vi "AnalysatorStringLaden.vi"(11 "Array (Eingang)":string[][](array[string])) -> (2 "string array":string[][](array[string]), 3 "Cluster Array (Ausgang)":T1[](array[typedef]))   [LabVIEW 2020, in "System Einstellungen V2.lvlib"]
uses:
  System Einstellungen V2.lvlib
  AnalysatorDefinition.ctl
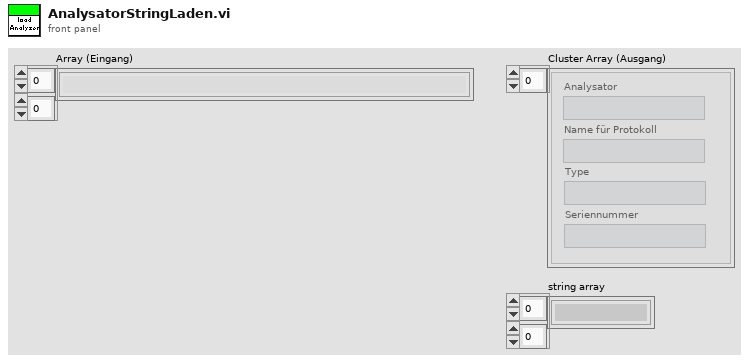
[diagram p1: front panel]
types:
  T1 = typedef "System Einstellungen V2.lvlib/AnalysatorDefinition.ctl" = cluster{"Analysator":string, "Name für Protokoll":string, "Type":string, "Seriennummer":string}
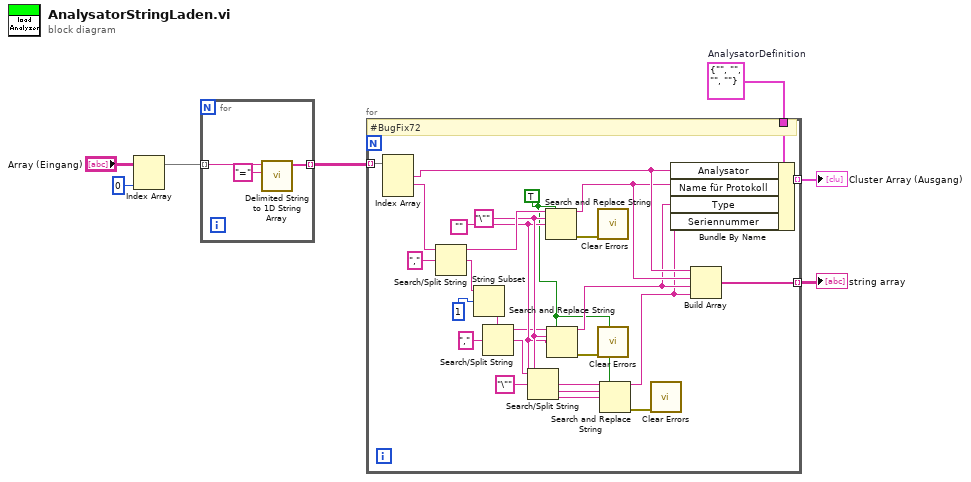
[diagram p0: block diagram]
diagram:
  w6 = T1 {"Analysator"="", "Name für Protokoll"="", "Type"="", "Seriennummer"=""}  # AnalysatorDefinition
  n1 = Index Array(array="Array (Eingang)", index (col)=0 ("Deaktivierter Index (Spalte)")) -> (element=w4:string[])  [unwired: 1 in]
  n2 = for {
    tunnel: w4 -> [w10] mode=indexing
    tunnel: [w8] -> w3 mode=indexing
    n3 = call <vilib>:"Delimited String to 1D String Array.vi"("delimiter"="=", "delimited string"=w10) -> ("string array"=w8:string[])  [unwired: 9 in]
  }
  n4 = for {
    tunnel: w3 -> [w34] mode=indexing
    tunnel: w6 -> [w35]
    tunnel: [w33] -> w7 mode=indexing
    tunnel: [w29] -> w2 mode=indexing
    w16 = ""
    w15 = TRUE ("Alle ersetzen? (F)")
    w17 = "\"" ("Such-String")
    # "#BugFix72"
    n5 = Index Array(array=w34) -> (element #1=w31:string, element #2=w28:string)  [unwired: 3 in, 1 out]
    n6 = Search/Split String(string=w28, search string/char (-)="," ("Such-String/-Zeichen (-)")) -> (substring before match=w26:string, match + rest of string=w24:string)  [unwired: 1 in, 1 out]
    n7 = String Subset(string=w24, offset (0)=1 ("Offset (0)")) -> (substring=w12:string)  [unwired: 1 in]
    n8 = Search/Split String(string=w12, search string/char (-)="," ("Such-String/-Zeichen (-)")) -> (substring before match=w14:string, match + rest of string=w20:string)  [unwired: 1 in, 1 out]
    n9 = Search/Split String(string=w20, search string/char (-)="\"" ("Such-String/-Zeichen (-)")) -> (match + rest of string=w18:string)  [unwired: 1 in, 2 out]
    n10 = Search and Replace String(replace all?=w15, input string=w26, search string=w17, replace string=w16) -> (result string=w30:string, error out=w32:errorcluster)  [unwired: 4 in, 2 out]
    n11 = Search and Replace String(replace all?=w15, input string=w14, search string=w17, replace string=w16) -> (result string=w22:string, error out=w23:errorcluster)  [unwired: 4 in, 2 out]
    n12 = call <vilib>:"Clear Errors.vi"("error in (no error)"=w32) -> ()  [unwired: 5 in, 2 out]
    n13 = call <vilib>:"Clear Errors.vi"("error in (no error)"=w23) -> ()  [unwired: 5 in, 2 out]
    n14 = Search and Replace String(replace all?=w15, input string=w18, search string=w17, replace string=w16) -> (result string=w13:string, error out=w19:errorcluster)  [unwired: 4 in, 2 out]
    n15 = call <vilib>:"Clear Errors.vi"("error in (no error)"=w19) -> ()  [unwired: 5 in, 2 out]
    n16 = Bundle By Name(cluster=w35, "Analysator"=w31, "Name für Protokoll"=w30, "Type"=w22, "Seriennummer"=w13) -> (w33:T1)
    n17 = Build Array(w31, w30, w22, w13) -> (w29:string[])
  }
  "Cluster Array (Ausgang)" <- w7
  "string array" <- w2
